vi "test-PID-input-output.vi"(8 "error in (no error)":errorcluster) -> (0 "error out":errorcluster, 3 "All Passed":bool)   [LabVIEW 2019]
uses:
  <vilib>/Rock Robotics/WPI/ThirdParty/JAS_Junk/TrajLib/PID_CONTROLLER.ctl
  <vilib>/Rock Robotics/WPI/ThirdParty/JAS_Junk/TrajLib/PIDController_NewPeriod.vi
  <vilib>/Rock Robotics/WPI/ThirdParty/JAS_Junk/TrajLib/PIDController_SetSetpoint.vi
  <vilib>/Rock Robotics/WPI/ThirdParty/JAS_Junk/TrajLib/PIDController_Calculate_PV.vi
  <vilib>/Rock Robotics/SystemInterfaces/NetworkCommunication/NetComm_UsageReport_report.vi
  <vilib>/Rock Robotics/WPI/ThirdParty/JAS_Junk/TrajLib/ControllerUtil_GetModulusError.vi
  <vilib>/Rock Robotics/WPI/ThirdParty/JAS_Junk/TrajLib/Util_LibraryGlobals.vi
  <vilib>/Rock Robotics/WPI/ThirdParty/JAS_Junk/TrajLib/Trajectory_Library.lvlib
panel:
  out "T3 Passed":bool
  out "T2 Passed":bool
  out "T1 Passed":bool
  out "T0 Passed":bool
  out "T0 PID CTRL":T1={"Kp"=0.0, "Ki"=0.0, "Kd"=0.0, "Period"=0.0, "Max_Integral"=0.0, "Min_Integral"=0.0, "Max_Input"=0.0, "Min_Input"=0.0, "Continuous"=FALSE, "PositionError"=0.0, "VelocityError"=0.0, "PrevError"=0.0, "TotalError"=0.0, "PositionTolerance"=0.0, "VelocityTolerance"=0.0, "SetPoint"=0.0, "Kf"=0.0, "Prev_Deriv"=0.0, "Prev_Deriv 2"=0.0, "DerivativeFilter"=FALSE, "Min_Output"=-9.99e+35, "Max_Output"=9.9e+35, "Prev_F_P"=0.0, "Prev_F_P_2"=0.0, "AntiWindupActive"=FALSE, "Measurement"=0.0} {"Measurement" format="%16_6e"; "Prev_F_P_2" format="%16_6e"; "Prev_F_P" format="%16_6e"; "Max_Output" format="%16_6e"; "Min_Output" format="%16_6e"; "Prev_Deriv 2" format="%16_6e"; "Prev_Deriv" format="%16_6e"; "Kf" format="%16_6e"; "SetPoint" format="%16_6e"; "VelocityTolerance" format="%16_6e"; "PositionTolerance" format="%16_6e"; "TotalError" format="%16_6e"; "PrevError" format="%16_6e"; "VelocityError" format="%16_6e"; "PositionError" format="%16_6e"; "Min_Input" format="%16_6e"; "Max_Input" format="%16_6e"; "Min_Integral" format="%16_6e"; "Max_Integral" format="%16_6e"; "Period" format="%16_6e"; "Kd" format="%16_6e"; "Ki" format="%16_6e"; "Kp" format="%16_6e"}
  out "T3 -- Output =":dbl
  out "T2 -- Output  = -0.01":dbl
  out "T1 -- Output  = -0.1":dbl
  out "T0 -- Output < 0":dbl
  # "PID Input Output"
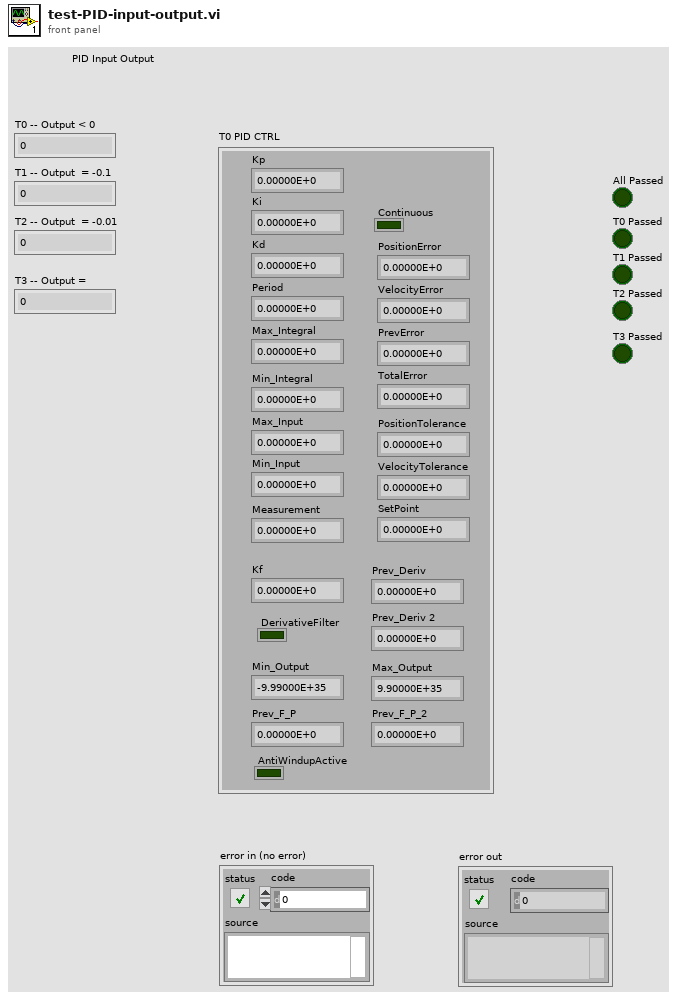
[diagram p1: front panel]
types:
  T1 = typedef "Trajectory_Library.lvlib/PID_CONTROLLER.ctl" = cluster{"Kp":dbl, "Ki":dbl, "Kd":dbl, "Period":dbl, "Max_Integral":dbl, "Min_Integral":dbl, "Max_Input":dbl, "Min_Input":dbl, "Continuous":bool, "PositionError":dbl, "VelocityError":dbl, "PrevError":dbl, "TotalError":dbl, "PositionTolerance":dbl, "VelocityTolerance":dbl, "SetPoint":dbl, "Kf":dbl, "Prev_Deriv":dbl, "Prev_Deriv 2":dbl, "DerivativeFilter":bool, "Min_Output":dbl, "Max_Output":dbl, "Prev_F_P":dbl, "Prev_F_P_2":dbl, "AntiWindupActive":bool, "Measurement":dbl}
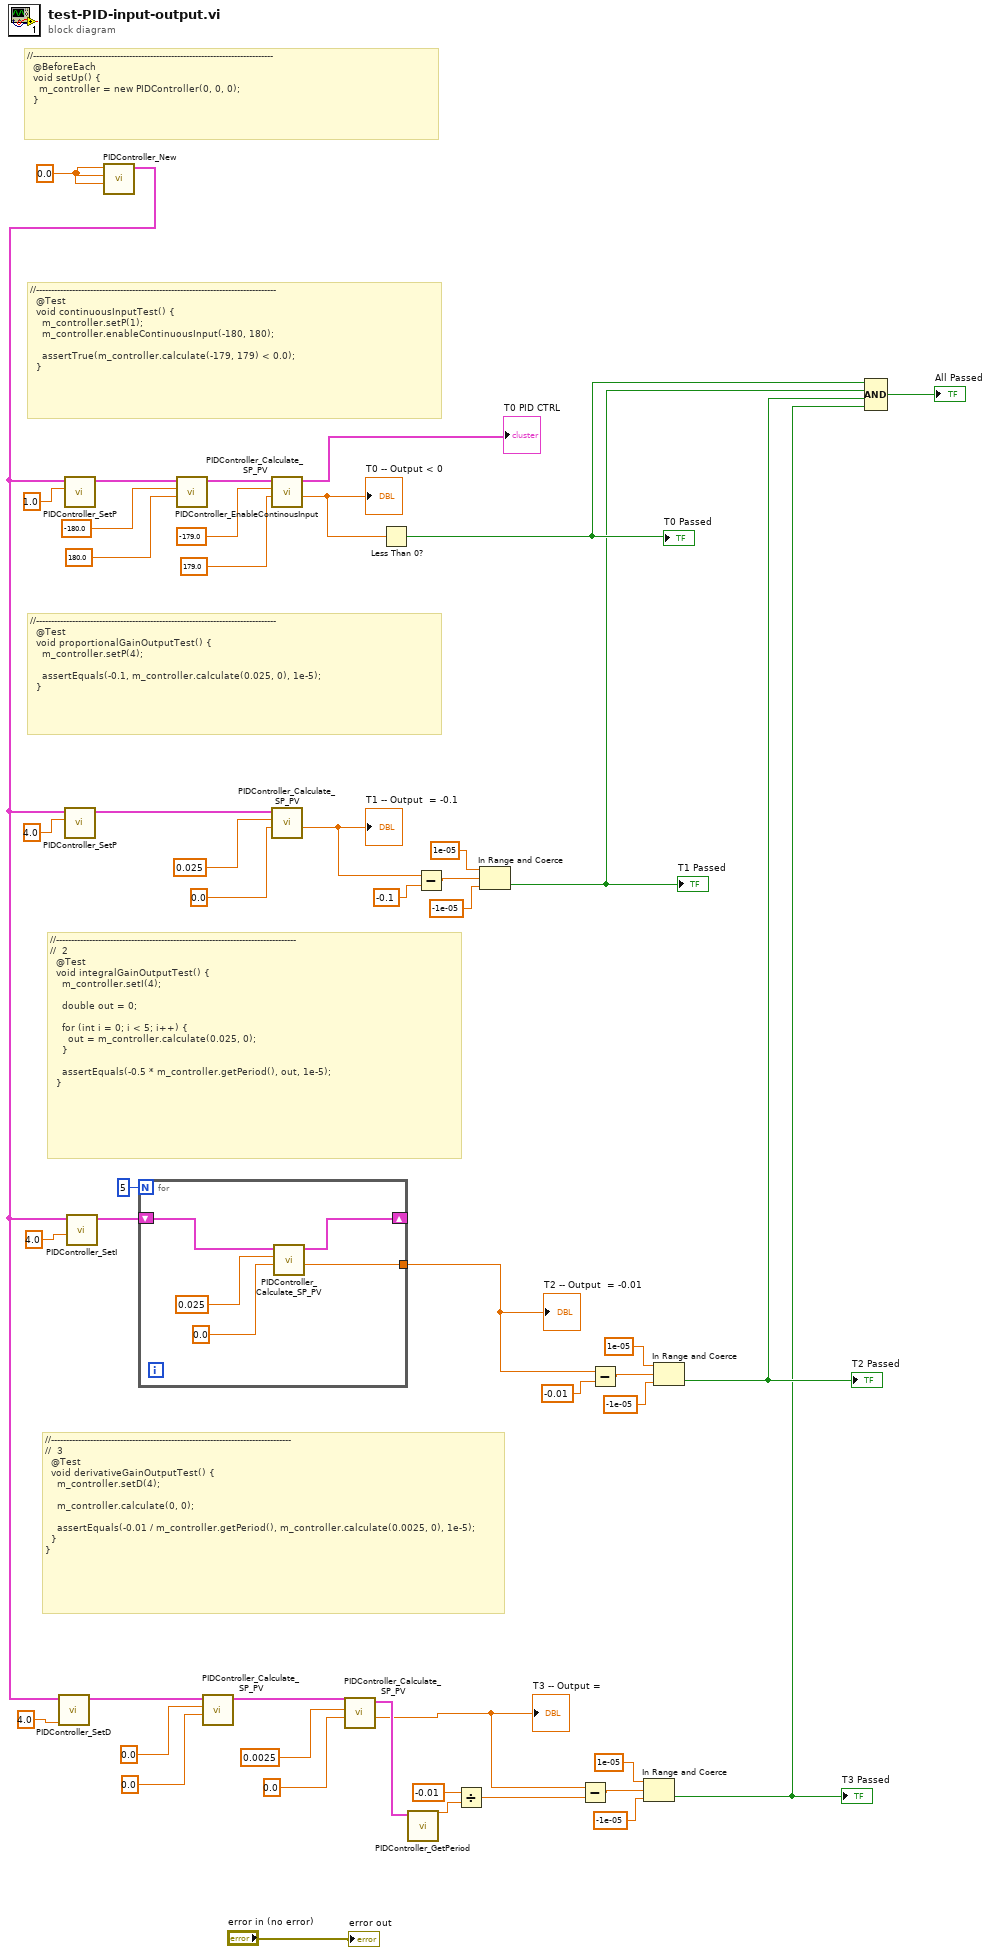
[diagram p0: block diagram]
diagram:
  w49 = 0.0 ("Kp")
  # "//--------------------------------------------------------------------------------\n//  3\n  @Test\n  void derivativeGainOutputTest() {\n    m_controller.setD(4);\n\n    m_controller.calculate(0, 0);\n\n    assertEquals(-0.01 / m_controller.getPeriod(), m_controller.calculate(0.0025, 0), 1e-5);\n  }\n}"
  # "//--------------------------------------------------------------------------------\n//  2\n  @Test\n  void integralGainOutputTest() {\n    m_controller.setI(4);\n\n    double out = 0;\n\n    for (int i = 0; i < 5; i++) {\n      out = m_controller.calculate(0.025, 0);\n    }\n\n    assertEquals(-0.5 * m_controller.getPeriod(), out, 1e-5);\n  }"
  # "//--------------------------------------------------------------------------------\n  @Test\n  void proportionalGainOutputTest() {\n    m_controller.setP(4);\n\n    assertEquals(-0.1, m_controller.calculate(0.025, 0), 1e-5);\n  }"
  # "//--------------------------------------------------------------------------------\n  @BeforeEach\n  void setUp() {\n    m_controller = new PIDController(0, 0, 0);\n  }"
  # "//--------------------------------------------------------------------------------\n  @Test\n  void continuousInputTest() {\n    m_controller.setP(1);\n    m_controller.enableContinuousInput(-180, 180);\n\n    assertTrue(m_controller.calculate(-179, 179) < 0.0);\n  }"
  n1 = call <vilib>:"PIDController_New.vi"("Kd"=w49, "Ki"=w49, "Kp"=w49) -> ("PID_CONTROLLER"=w30:T1)  [unwired: 8 in]
  n2 = call <vilib>:"PIDController_SetD.vi"("Kd"=4.0 ("Kp"), "in PID_CONTROLLER"=w30) -> ("out PID_CONTROLLER"=w33:T1)  [unwired: 9 in]
  n3 = call <vilib>:"PIDController_SetP.vi"("Kp"=1.0, "in PID_CONTROLLER"=w30) -> ("out PID_CONTROLLER"=w47:T1)  [unwired: 9 in]
  n4 = call <vilib>:"PIDController_SetP.vi"("Kp"=4.0, "in PID_CONTROLLER"=w30) -> ("out PID_CONTROLLER"=w38:T1)  [unwired: 9 in]
  n5 = call <vilib>:"PIDController_SetI.vi"("Ki"=4.0 ("Kp"), "in PID_CONTROLLER"=w30) -> ("out PID_CONTROLLER"=w36:T1)  [unwired: 9 in]
  n6 = for {
    N: 5 -> [_]
    tunnel: [w52] -> w15
    shift-right: [w50] -> _
    shift-left: w36 -> [w51]
    n7 = call <vilib>:"PIDController_Calculate_SP_PV.vi"("SP-SetPoint"=0.0, "PV-Measurement"=0.025, "in PID_CONTROLLER"=w51) -> ("CO-ControlOutput"=w52:dbl, "out PID_CONTROLLER"=w50:T1)  [unwired: 7 in]
  }
  "T2 -- Output  = -0.01" <- w15
  n8 = call <vilib>:"PIDController_EnableContinousInput.vi"("MaxInput"=180.0, "MinInput"=-180.0, "in PID_CONTROLLER"=w47) -> ("out PID_CONTROLLER"=w44:T1)  [unwired: 8 in]
  n9 = call <vilib>:"PIDController_Calculate_SP_PV.vi"("SP-SetPoint"=0.0, "PV-Measurement"=0.0, "in PID_CONTROLLER"=w33) -> ("out PID_CONTROLLER"=w27:T1)  [unwired: 7 in, 1 out]
  n10 = call <vilib>:"PIDController_Calculate_SP_PV.vi"("SP-SetPoint"=179.0, "PV-Measurement"=-179.0, "in PID_CONTROLLER"=w44) -> ("CO-ControlOutput"=w25:dbl, "out PID_CONTROLLER"=→"T0 PID CTRL":T1)  [unwired: 7 in]
  "T0 -- Output < 0" <- w25
  n11 = call <vilib>:"PIDController_Calculate_SP_PV.vi"("SP-SetPoint"=0.0, "PV-Measurement"=0.025, "in PID_CONTROLLER"=w38) -> ("CO-ControlOutput"=w23:dbl)  [unwired: 7 in, 1 out]
  "T1 -- Output  = -0.1" <- w23
  n12 = call <vilib>:"PIDController_Calculate_SP_PV.vi"("SP-SetPoint"=0.0, "PV-Measurement"=0.0025, "in PID_CONTROLLER"=w27) -> ("CO-ControlOutput"=w7:dbl, "out PID_CONTROLLER"=w14:T1)  [unwired: 7 in]
  "T3 -- Output =" <- w7
  n13 = Less Than 0?(x=w25) -> (x < 0?=w6:bool)
  "T0 Passed" <- w6
  n14 = call <vilib>:"PIDController_GetPeriod.vi"("in PID_CONTROLLER"=w14) -> ("Period"=w13:dbl)  [unwired: 10 in]
  n15 = Subtract(x=w23, y=-0.1) -> (x-y=w20:dbl)
  n16 = Divide(x=-0.01, y=w13) -> (x/y=w8:dbl)
  n17 = In Range and Coerce(upper limit=1e-05, x=w20, lower limit=-1e-05 ("upper limit")) -> (In Range?=w5:bool)  [unwired: 1 out]
  "T1 Passed" <- w5
  n18 = Subtract(x=w7, y=w8) -> (x-y=w10:dbl)
  n19 = Subtract(x=w15, y=-0.01) -> (x-y=w17:dbl)
  n20 = In Range and Coerce(upper limit=1e-05, x=w10, lower limit=-1e-05 ("upper limit")) -> (In Range?=w2:bool)  [unwired: 1 out]
  "T3 Passed" <- w2
  n21 = In Range and Coerce(upper limit=1e-05, x=w17, lower limit=-1e-05 ("upper limit")) -> (In Range?=w3:bool)  [unwired: 1 out]
  "T2 Passed" <- w3
  n22 = Compound Arithmetic op=AND(w6, w5, w3, w2) -> (→"All Passed":bool)
  "error out" <- "error in (no error)"
